vi "stayAwayBall.vi"(0 "object in":refnum<class "DefenderAreaRole.lvclass">, 2 "Robot":refnum<class "Robot.lvclass">, 4 "Ball":refnum<class "Ball.lvclass">, 5 "error in (no error)":errorcluster) -> (14 "object out":refnum<class "DefenderAreaRole.lvclass">, 18 "Robot out":refnum<class "Robot.lvclass">, 19 "error out":errorcluster)   [LabVIEW 2024, in "DefenderAreaRole.lvclass"]
uses:
  DefenderAreaRole.lvclass
  Robot_class/Robot.lvclass
  Ball_class/Ball.lvclass
  C:/Users/ROBOIME2/Documents/SSL ROBOIME/SSL_AI/Object_class/Object.lvclass
  Robot_class/Robot.lvclass/Robot.ctl
  Object_class/Object.lvclass/Object.ctl
  <vilib>/Analysis/baseanly.llb/Unit Vector (DBL).vi
  Object_class/Read position(x,y).vi
  Robot_class/Read dest_x.vi
  Robot_class/Read dest_y.vi
  Robot_class/Write dest_x.vi
  Robot_class/Write dest_y.vi
  <vilib>/Analysis/NI_AALBase.lvlib
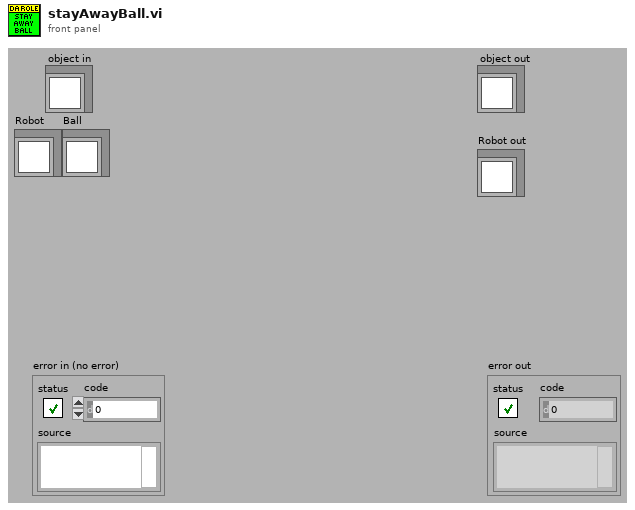
[diagram p1: front panel]
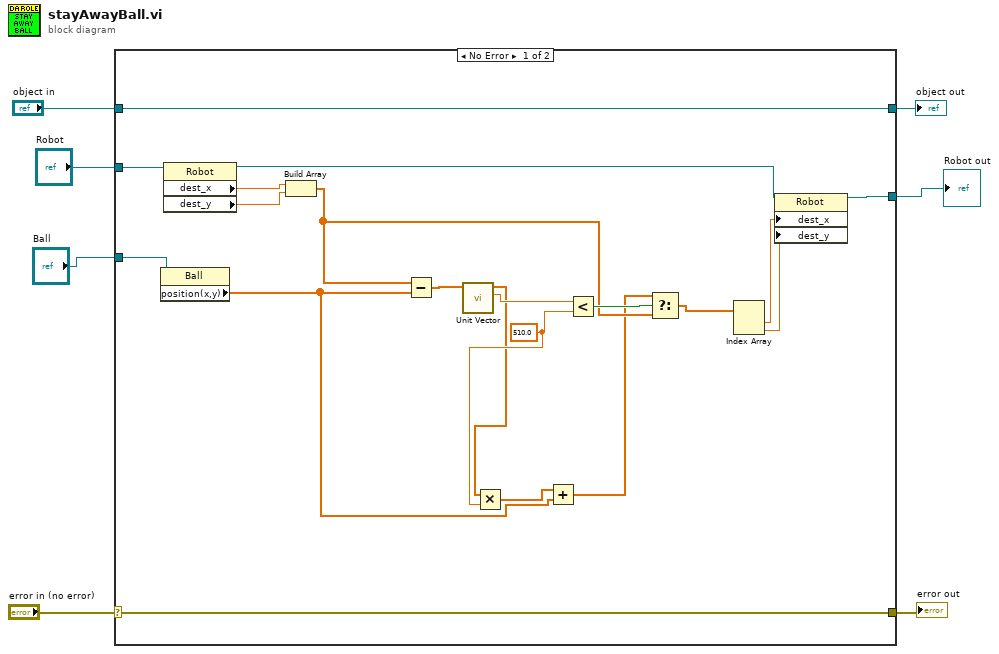
[diagram p0: block diagram]
diagram:
  n1 = case shown="No Error" "error in (no error)" {
    selector: "error in (no error)" -> [w26 w29]
    tunnel: [w26 w29] -> w6
    tunnel: [w27 w28] -> w4
    tunnel: "object in" -> [w27 w28]
    tunnel: "Robot" -> [w25 _]
    tunnel: "Ball" -> [w24 _]
    tunnel: [w18 _] -> w1
    frame No Error {
      w12 = 510.0 ("y")
      n2 = property class="Ball"(reference=w24) -> ("position(x,y)"=w9:dbl[])  [unwired: 1 in, 2 out]
      n3 = property class="Robot"(reference=w25) -> (reference out=w17:refnum<class "Robot.lvclass">, "dest_x"=w23:dbl, "dest_y"=w22:dbl)  [unwired: 1 in, 1 out]
      n4 = Build Array(w23, w22) -> (w15:dbl[])
      n5 = Subtract(x=w15, y=w9) -> (x-y=w21:dbl[])
      n6 = call-poly <vilib>:"Unit Vector.vi"("Input Vector"=w21) -> ("norm"=w20:dbl, "Unit Vector"=w11:dbl[])  [unwired: 8 in, 1 out]
      n7 = Multiply(x=w11, y=w12) -> (x*y=w10:dbl[])
      n8 = Add(x=w10, y=w9) -> (x+y=w8:dbl[])
      n9 = Less?(x=w20, y=w12) -> (x < y?=w19:bool)
      n10 = Select(t=w8, s=w19, f=w15) -> (s? t:f=w16:dbl[])
      n11 = Index Array(array=w16) -> (element #1=w14:dbl, element #2=w13:dbl)  [unwired: 2 in]
      n12 = property class="Robot"(reference=w17, "dest_x"=w14, "dest_y"=w13) -> (reference out=w18:refnum<class "Robot.lvclass">)  [unwired: 1 in, 1 out]
    }
    frame Error {
    }
  }
  "error out" <- w6
  "object out" <- w4
  "Robot out" <- w1
